vi "Results_Row_Per_Channel.vi"(0 "Analysis_info_cluster":T1={"Colour"=0, "Inst type"=enum."Pitot-static tube", "Inst name"="Manometer voltage", "Symbol"="U", "Code name"="", "Extra Info"="U", "Inst Array"=enum."PWA", "Extra Titles"=[], "Extra Values"=[], "U"=0.0, "u^2"=0.0, "u^3"=0.0, "u^4"=0.0, "Skew_u"=0.0, "Kurt_u"=0.0, "Sd Error in Mean"=0.0, "% u'/U"=0.0, "X"=0.0, "Y"=0.0, "Z"=0.0, "Timescale integral to 25%"=0.0, "Sd Error in Variance"=0.0, "Calib File"=path "", "Calib Constants"=[], "Output Position"=FALSE, "Full Stats"=FALSE, "Av Sampling Rate"=0.0, "Av No of Samples"=0.0, "Total Meas Time (s)"=0.0, "ADAM Ch Name"=""} {"Sd Error in Variance" format="%.2f"; "Skew_u" format="%.2f"; "% u'/U" format="%.2f"; "Sd Error in Mean" format="%.2f"; "Kurt_u" format="%.2f"; "u^4" format="%.2f"; "u^3" format="%.2f"; "U" format="%.2f"; "u^2" format="%.2f"}) -> (1 "Channel Names":string[](array[string]), 2 "Channel Values":string[](array[string]))   [LabVIEW 2014]
uses:
  Controls/Analysis_info_cluster.ctl
  Controls/Inst_type.ctl
  Controls/Instrument_Array.ctl
  Controls/Post_Process.ctl
  Globals/Trav_pos_global.vi
  Acquisition/PWA/PWAtasksGLOBAL.vi
  Globals/Meas_global.vi
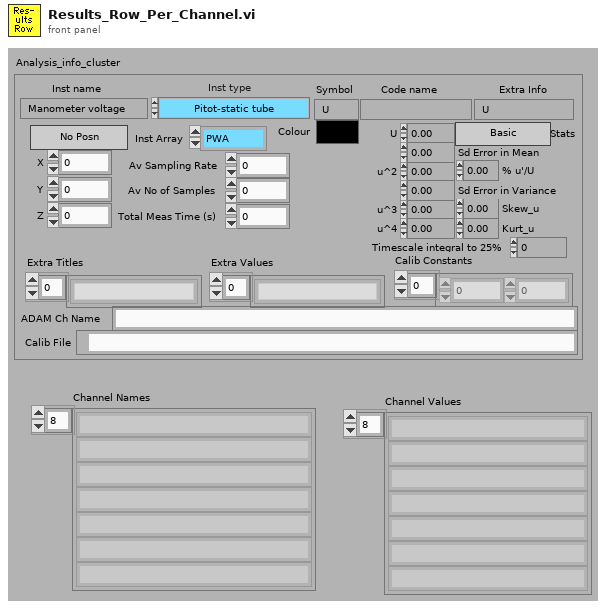
[diagram p1: front panel]
types:
  T1 = typedef "Analysis_info_cluster.ctl" = cluster{"Colour":u32, "Inst type":T2, "Inst name":string, "Symbol":string, "Code name":string, "Extra Info":string, "Inst Array":T3, "Extra Titles":string[], "Extra Values":string[], "U":dbl, "u^2":dbl, "u^3":dbl, "u^4":dbl, "Skew_u":dbl, "Kurt_u":dbl, "Sd Error in Mean":dbl, "% u'/U":dbl, "X":dbl, "Y":dbl, "Z":dbl, "Timescale integral to 25%":dbl, "Sd Error in Variance":dbl, "Calib File":path, "Calib Constants":dbl[], "Output Position":bool, "Full Stats":bool, "Av Sampling Rate":dbl, "Av No of Samples":dbl, "Total Meas Time (s)":dbl, "ADAM Ch Name":string}
  T2 = typedef "Inst_type.ctl" = enum16{"Propeller anemometer", "Raw voltage", "Pressure Transducer", "Pitot-static tube", "Preston tube", "Hot wire", "Cross wire 1", "Cross wire 2", "Generic Linear", "Generic Polynomial", "Generic BackPoly", "Fast FID", "Thermocouple", "Cold wire", "Pulsed Wire", "LDA Vel", "LDA Tran time", "LDA Arr time", "Microphone"}
  T3 = typedef "Instrument_Array.ctl" = enum16{"PWA", "LDA", "Analogue"}
  T4 = enum16{"Mean only", "2nd Order Stats", "4th Order Stats"}
  T5 = typedef "Post_Process.ctl" = enum16{"Take New Data", "Post Process Raw Data File"}
  T6 = typedef "Tunnel_Coordinates.ctl" = enum16{"Work in Tunnel Coordinates", "Work in Model Coordinates"}
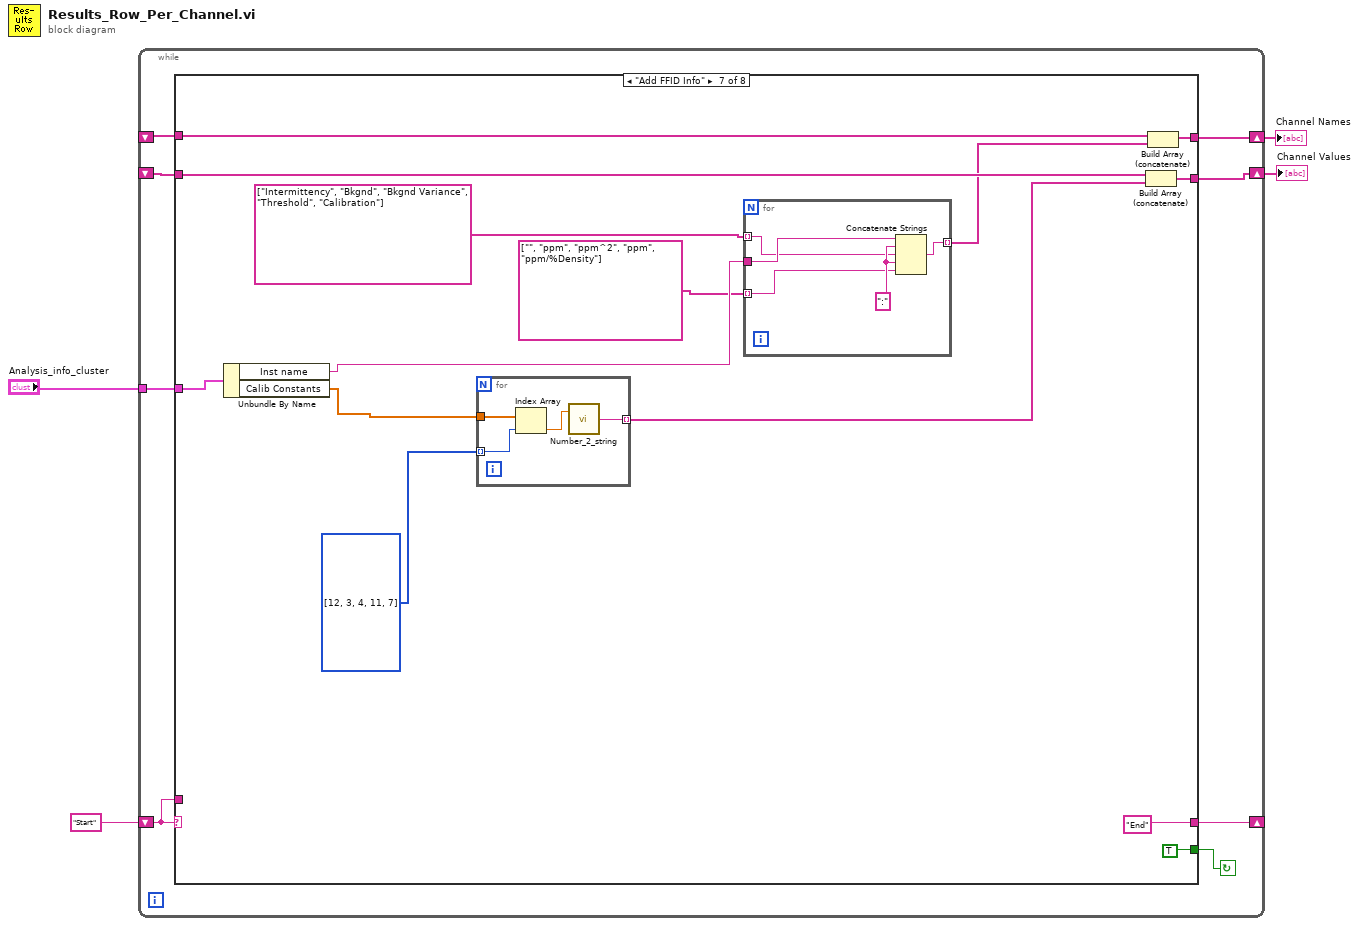
[diagram p0: block diagram]
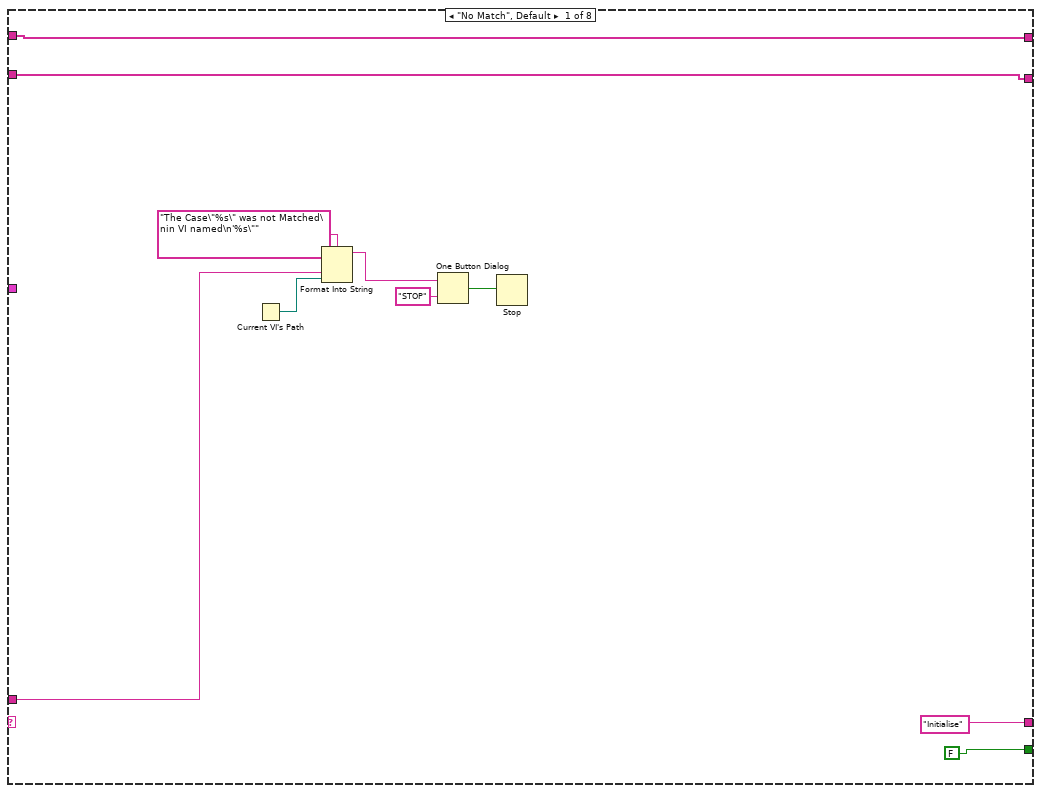
[diagram p2: hidden frame]
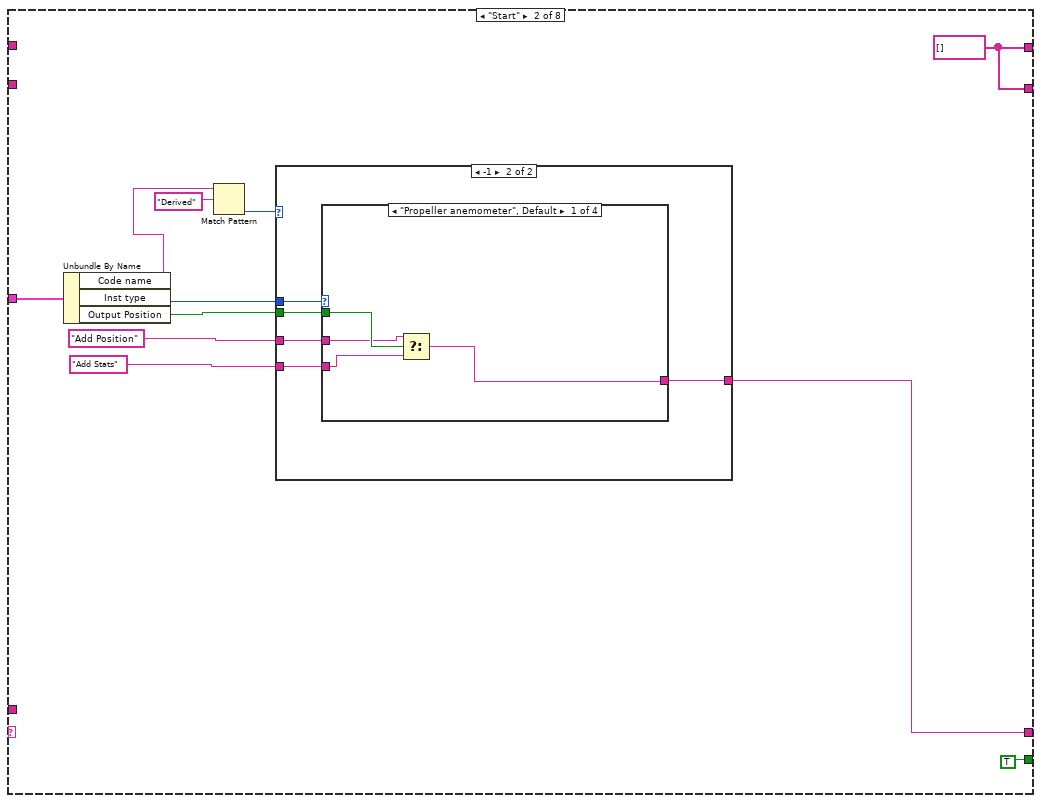
[diagram p3: hidden frame]
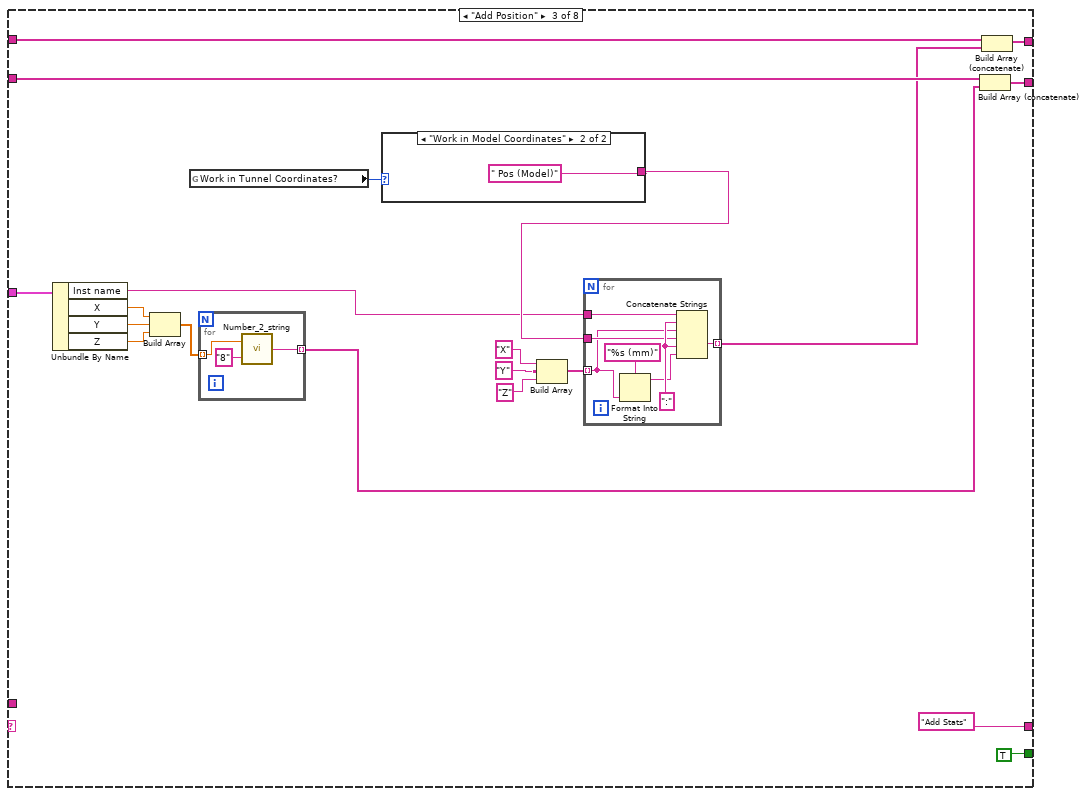
[diagram p8: hidden frame]
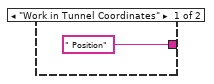
[diagram p9: hidden frame]
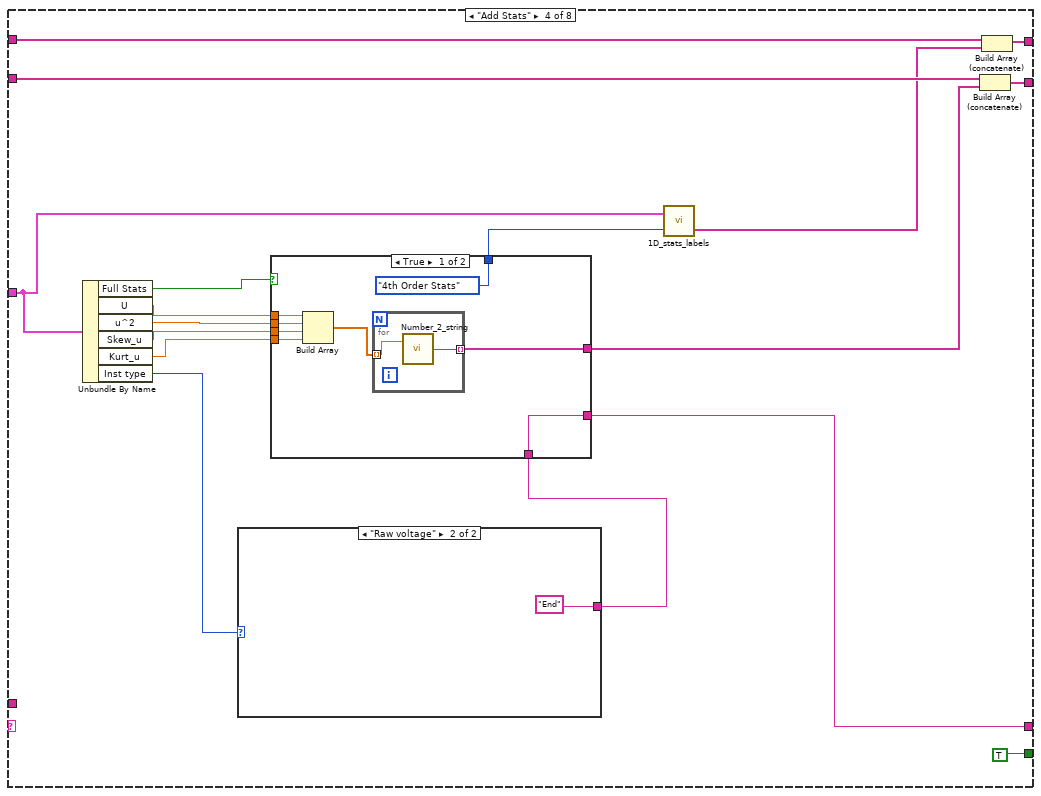
[diagram p10: hidden frame]
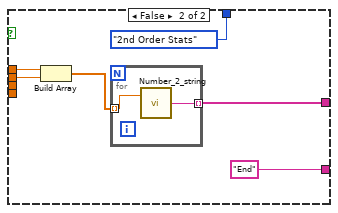
[diagram p11: hidden frame]
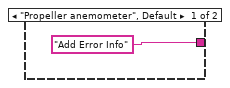
[diagram p12: hidden frame]
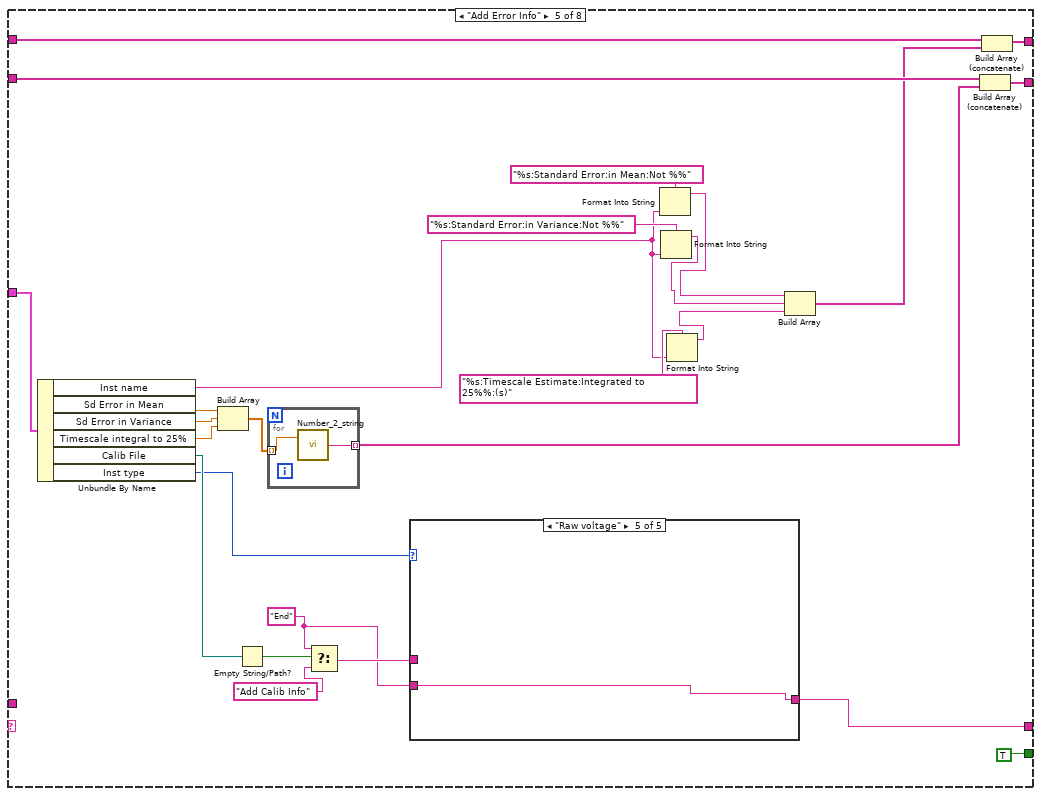
[diagram p13: hidden frame]
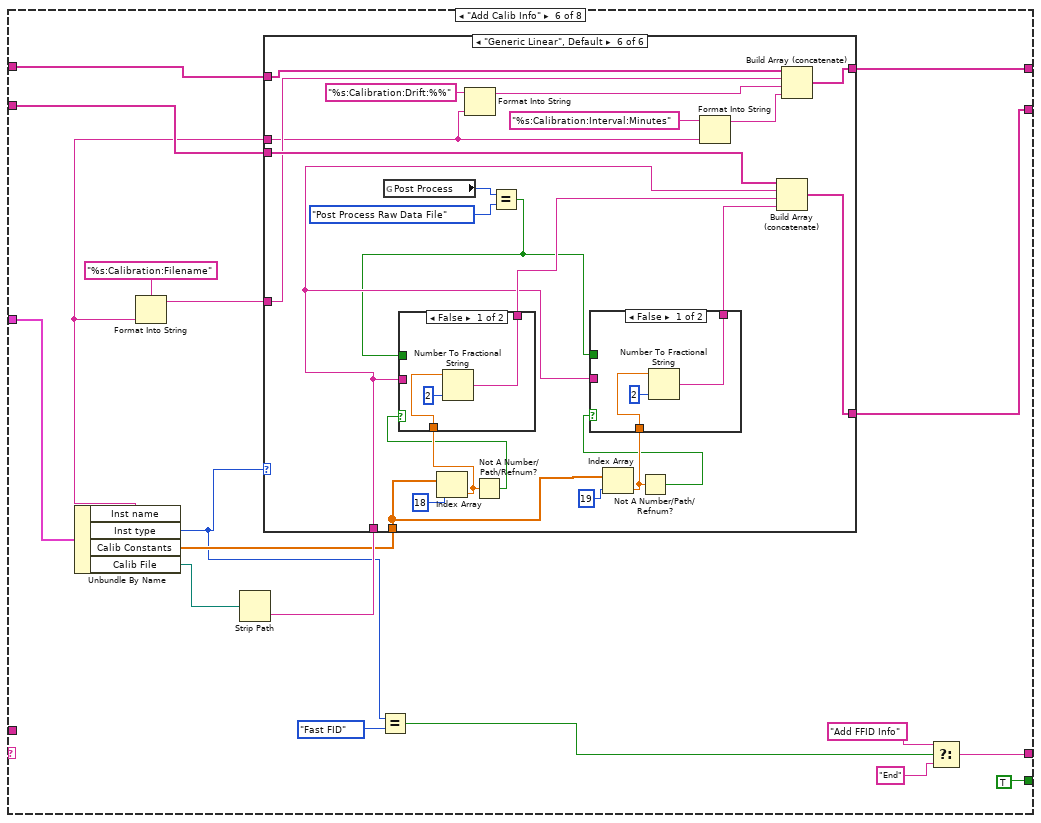
[diagram p18: hidden frame]
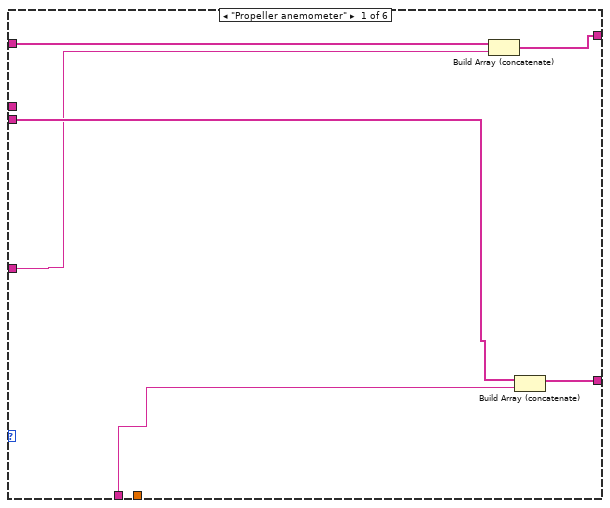
[diagram p19: hidden frame]
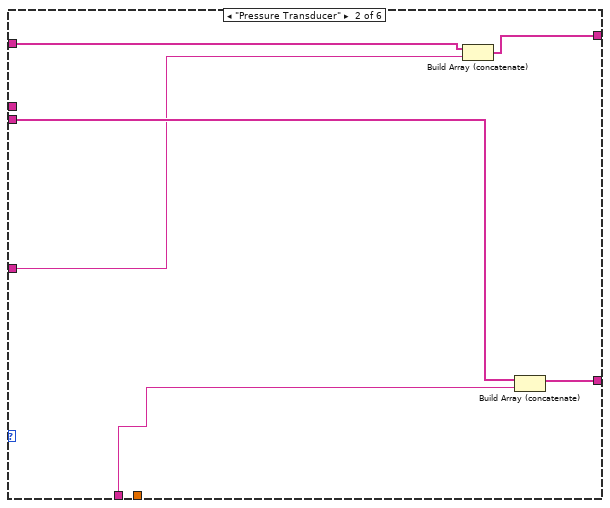
[diagram p20: hidden frame]
diagram:
  n1 = while {
    shift-left: "Start" -> [w10]
    shift-right: [w11] -> _
    shift-right: [w5] -> w1
    shift-left: _ -> [w6]
    shift-right: [w8] -> w2
    shift-left: _ -> [w7]
    tunnel: "Analysis_info_cluster" -> [w9]
    stop <- w12 continue-if-true
    n2 = case shown="\"Add FFID Info\"" w10 {
      tunnel: [FALSE TRUE TRUE TRUE TRUE TRUE TRUE FALSE] -> w12
      tunnel: ["Initialise" w30 "Add Stats" w81 w118 w151 "End" "End"] -> w11
      tunnel: w10 -> [w18 _ _ _ _ _ _ _]
      tunnel: w9 -> [_ w32 w58 w86 w133 w165 w247 w268]
      tunnel: [w13 w28 w51 w91 w137 w161 w251 w262] -> w8
      tunnel: w7 -> [w13 _ w50 w90 w136 w163 w250 w265]
      tunnel: w6 -> [w14 _ w49 w89 w135 w158 w249 w267]
      tunnel: [w14 w28 w48 w88 w134 w156 w248 w263] -> w5
      frame "No Match", Default {
        n3 = Current VI's Path() -> (path=w17:path)
        n4 = Format Into String(format string="The Case\"%s\" was not Matched\nin VI named\n'%s\"" ("Format String"), w18, w17) -> (resulting string=w21:string)  [unwired: 2 in, 1 out]
        n5 = One Button Dialog(message=w21, button name ("OK")="STOP") -> (true=w19:bool)
        n6 = Stop(stop? (T)=w19) -> ()
      }
      frame "Start" {
        w28 = string[] []
        n7 = Unbundle By Name(w32) -> ("Code name"=w25:string, "Inst type"=w31:T2, "Output Position"=w23:bool)
        n8 = Match Pattern(string=w25, regular expression="Derived") -> (offset past match=w24:i32)  [unwired: 1 in, 3 out]
        n9 = case shown="-1" w24 {
          tunnel: w31 -> [_ w39]
          tunnel: [w34 w38] -> w30
          tunnel: "Add Position" -> [_ w37]
          tunnel: "Add Stats" -> [w34 w36]
          tunnel: w23 -> [_ w35]
          frame 0, Default {
          }
          frame -1 {
            n10 = case shown="\"Propeller anemometer\", Default" w39 {
              tunnel: [w40 w44 w45 w46] -> w38
              tunnel: w37 -> [w42 _ _ _]
              tunnel: w36 -> [w41 w44 w45 w46]
              tunnel: w35 -> [w43 _ _ _]
              frame "Propeller anemometer", Default {
                n11 = Select(t=w42, s=w43, f=w41) -> (s? t:f=w40:string)
              }
              frame "Cross wire 2" {
              }
              frame "LDA Tran time" {
              }
              frame "LDA Arr time" {
              }
            }
          }
        }
      }
      frame "Add Position" {
        n12 = Unbundle By Name(w58) -> ("Inst name"=w57:string, "X"=w56:dbl, "Y"=w55:dbl, "Z"=w54:dbl)
        n13 = Build Array(w56, w55, w54) -> (w53:dbl[])
        n14 = global read "Trav_pos_global.vi" "Work in Tunnel Coordinates?"() -> (w64:T6)
        n15 = for {
          tunnel: w53 -> [w69] mode=indexing
          tunnel: [w68] -> w52 mode=indexing
          n16 = call "Number_2_string.vi"("precision"="8", "number"=w69) -> ("String"=w68:string)
        }
        n17 = case shown="\"Work in Model Coordinates\"" w64 {
          tunnel: [" Position" " Pos (Model)"] -> w59
          frame "Work in Tunnel Coordinates" {
          }
          frame "Work in Model Coordinates" {
          }
        }
        n18 = Build Array("X", "Y", "Z") -> (w63:string[])
        n19 = for {
          tunnel: w63 -> [w72] mode=indexing
          tunnel: w57 -> [w76]
          tunnel: [w74] -> w47 mode=indexing
          tunnel: w59 -> [w73]
          w75 = ":" ("Substring")
          n20 = Format Into String(format string="%s (mm)", w72) -> (resulting string=w70:string)  [unwired: 2 in, 1 out]
          n21 = Concatenate Strings(w76, w75, w72, w73, w75, w70) -> (w74:string)
        }
        n22 = Build Array (concatenate)(w50, w52) -> (w51:string[])
        n23 = Build Array (concatenate)(w49, w47) -> (w48:string[])
      }
      frame "Add Stats" {
        n24 = Unbundle By Name(w86) -> ("Full Stats"=w79:bool, "U"=w95:dbl, "u^2"=w94:dbl, "Skew_u"=w93:dbl, "Kurt_u"=w87:dbl, "Inst type"=w84:T2)
        n25 = case shown="\"Raw voltage\"" w84 {
          tunnel: ["Add Error Info" "End"] -> w80
          frame "Propeller anemometer", Default {
          }
          frame "Raw voltage" {
          }
        }
        n26 = case shown="True" w79 {
          tunnel: w95 -> [w103 w111]
          tunnel: w94 -> [w102 w110]
          tunnel: w93 -> [w101 _]
          tunnel: [w99 w108] -> w92
          tunnel: w87 -> [w98 _]
          tunnel: [T4."4th Order Stats" ("Mode selector") T4."2nd Order Stats" ("Mode selector")] -> w82
          tunnel: [w96 "End"] -> w81
          tunnel: w80 -> [w96 _]
          frame True {
            n27 = Build Array(w103, w102, w101, w98) -> (w100:dbl[])
            n28 = for {
              tunnel: w100 -> [w105] mode=indexing
              tunnel: [w104] -> w99 mode=indexing
              n29 = call "Number_2_string.vi"("number"=w105) -> ("String"=w104:string)  [unwired: 1 in]
            }
          }
          frame False {
            n30 = Build Array(w111, w110) -> (w109:dbl[])
            n31 = for {
              tunnel: w109 -> [w113] mode=indexing
              tunnel: [w112] -> w108 mode=indexing
              n32 = call "Number_2_string.vi"("number"=w113) -> ("String"=w112:string)  [unwired: 1 in]
            }
          }
        }
        n33 = call "1D_stats_labels.vi"("Mode selector"=w82, "Analysis Info Cluster"=w86) -> ("Output"=w85:string[])  [unwired: 1 in]
        n34 = Build Array (concatenate)(w90, w92) -> (w91:string[])
        n35 = Build Array (concatenate)(w89, w85) -> (w88:string[])
      }
      frame "Add Error Info" {
        w116 = "End"
        n36 = Unbundle By Name(w133) -> ("Inst name"=w126:string, "Sd Error in Mean"=w140:dbl, "Sd Error in Variance"=w124:dbl, "Timescale integral to 25%"=w123:dbl, "Calib File"=w122:path, "Inst type"=w117:T2)
        n37 = Build Array(w140, w124, w123) -> (w139:dbl[])
        n38 = Empty String/Path?(string/path=w122) -> (empty?=w121:bool)
        n39 = for {
          tunnel: w139 -> [w148] mode=indexing
          tunnel: [w147] -> w138 mode=indexing
          n40 = call "Number_2_string.vi"("number"=w148) -> ("String"=w147:string)  [unwired: 1 in]
        }
        n41 = Select(t=w116, s=w121, f="Add Calib Info") -> (s? t:f=w119:string)
        n42 = case shown="\"Raw voltage\"" w117 {
          tunnel: [w142 w143 w144 w145 w146] -> w118
          tunnel: w119 -> [w142 _ _ _ _]
          tunnel: w116 -> [_ w143 w144 w145 w146]
          frame "Propeller anemometer", Default {
          }
          frame "Cross wire 2" {
          }
          frame "LDA Tran time" {
          }
          frame "LDA Arr time" {
          }
          frame "Raw voltage" {
          }
        }
        n43 = Format Into String(format string="%s:Standard Error:in Mean:Not %%", w126) -> (resulting string=w128:string)  [unwired: 2 in, 1 out]
        n44 = Format Into String(format string="%s:Standard Error:in Variance:Not %%", w126) -> (resulting string=w130:string)  [unwired: 2 in, 1 out]
        n45 = Format Into String(format string="%s:Timescale Estimate:Integrated to 25%%:(s)", w126) -> (resulting string=w132:string)  [unwired: 2 in, 1 out]
        n46 = Build Array(w128, w130, w132) -> (w125:string[])
        n47 = Build Array (concatenate)(w136, w138) -> (w137:string[])
        n48 = Build Array (concatenate)(w135, w125) -> (w134:string[])
      }
      frame "Add Calib Info" {
        n49 = Unbundle By Name(w165) -> ("Inst name"=w155:string, "Inst type"=w154:T2, "Calib Constants"=w160:dbl[], "Calib File"=w164:path)
        n50 = Format Into String(format string="%s:Calibration:Filename" ("Format String"), w155) -> (resulting string=w157:string)  [unwired: 2 in, 1 out]
        n51 = Strip Path(path=w164) -> (name=w162:string)  [unwired: 1 out]
        n52 = case shown="\"Generic Linear\", Default" w154 {
          tunnel: [w172 w177 w183 w189 w196 w219] -> w161
          tunnel: w163 -> [w170 w178 w184 w190 w197 w220]
          tunnel: w162 -> [w171 w176 w182 w188 _ w213]
          tunnel: w160 -> [_ _ _ _ _ w212]
          tunnel: w158 -> [w169 w175 w181 w187 w193 w205]
          tunnel: w157 -> [w167 w174 w179 w186 w191 w204]
          tunnel: [w168 w173 w180 w185 w192 w199] -> w156
          tunnel: w155 -> [_ _ _ _ _ w198]
          frame "Propeller anemometer" {
            n53 = Build Array (concatenate)(w169, w167) -> (w168:string[])
            n54 = Build Array (concatenate)(w170, w171) -> (w172:string[])
          }
          frame "Pressure Transducer" {
            n55 = Build Array (concatenate)(w175, w174) -> (w173:string[])
            n56 = Build Array (concatenate)(w178, w176) -> (w177:string[])
          }
          frame "Pitot-static tube" {
            n57 = Build Array (concatenate)(w181, w179) -> (w180:string[])
            n58 = Build Array (concatenate)(w184, w182) -> (w183:string[])
          }
          frame "Preston tube" {
            n59 = Build Array (concatenate)(w190, w188) -> (w189:string[])
            n60 = Build Array (concatenate)(w187, w186) -> (w185:string[])
          }
          frame "Pulsed Wire" {
            n61 = global read "PWAtasksGLOBAL.vi" "PWA Calib. File Path"() -> (w195:path)
            n62 = Strip Path(path=w195) -> (name=w194:string)  [unwired: 1 out]
            n63 = Build Array (concatenate)(w193, w191) -> (w192:string[])
            n64 = Build Array (concatenate)(w197, w194) -> (w196:string[])
          }
          frame "Generic Linear", Default {
            n65 = global read "Meas_global.vi" "Post Process"() -> (w215:T5)
            n66 = Index Array(array=w212, index=18 ("Index")) -> (element=w218:dbl)
            n67 = Format Into String(format string="%s:Calibration:Drift:%%" ("Format String"), w198) -> (resulting string=w201:string)  [unwired: 2 in, 1 out]
            n68 = Not A Number/Path/Refnum?(number/path/refnum=w218) -> (NaN/Path/Refnum?=w217:bool)
            n69 = Equal?(x=w215, y=Post_Process."Post Process Raw Data File" ("Post Process")) -> (x = y?=w208:bool)
            n70 = case shown="False" w217 {
              tunnel: [w230 w235] -> w214
              tunnel: w218 -> [w231 _]
              tunnel: w208 -> [_ w237]
              tunnel: w213 -> [_ w234]
              frame False {
                n71 = Number To Fractional String(number=w231, precision (6)=i16 2) -> (F-format string=w230:string)  [unwired: 2 out]
              }
              frame True {
                n72 = Concatenate Strings(w234, "_Drift_Place_Holder" ("Substring")) -> (w236:string)
                n73 = Select(t="No Info", s=w237, f=w236) -> (s? t:f=w235:string)
              }
            }
            n74 = Index Array(array=w212, index=19 ("Index")) -> (element=w211:dbl)
            n75 = Not A Number/Path/Refnum?(number/path/refnum=w211) -> (NaN/Path/Refnum?=w210:bool)
            n76 = case shown="False" w210 {
              tunnel: [w221 w226] -> w209
              tunnel: w211 -> [w222 _]
              tunnel: w208 -> [_ w228]
              tunnel: w213 -> [_ w225]
              frame False {
                n77 = Number To Fractional String(number=w222, precision (6)=i16 2) -> (F-format string=w221:string)  [unwired: 2 out]
              }
              frame True {
                n78 = Concatenate Strings(w225, "_Interval_Place_Holder" ("Substring")) -> (w227:string)
                n79 = Select(t="No Info", s=w228, f=w227) -> (s? t:f=w226:string)
              }
            }
            n80 = Format Into String(format string="%s:Calibration:Interval:Minutes" ("Format String"), w198) -> (resulting string=w200:string)  [unwired: 2 in, 1 out]
            n81 = Build Array (concatenate)(w220, w213, w214, w209) -> (w219:string[])
            n82 = Build Array (concatenate)(w205, w204, w201, w200) -> (w199:string[])
          }
        }
        n83 = Equal?(x=w154, y=Inst_type."Fast FID" ("Inst type")) -> (x = y?=w153:bool)
        n84 = Select(t="Add FFID Info", s=w153, f="End") -> (s? t:f=w151:string)
      }
      frame "Add FFID Info" {
        n85 = Unbundle By Name(w247) -> ("Inst name"=w242:string, "Calib Constants"=w245:dbl[])
        n86 = for {
          tunnel: w245 -> [w261]
          tunnel: i32[] [12, 3, 4, 11, 7] ("Calib Constants") -> [w260] mode=indexing
          tunnel: [w258] -> w243 mode=indexing
          n87 = Index Array(array=w261, index=w260) -> (element=w259:dbl)
          n88 = call "Number_2_string.vi"("number"=w259) -> ("String"=w258:string)  [unwired: 1 in]
        }
        n89 = for {
          tunnel: string[] ["Intermittency", "Bkgnd", "Bkgnd Variance", "Threshold", "Calibration"] ("appended array") -> [w254] mode=indexing
          tunnel: w242 -> [w255]
          tunnel: [w256] -> w241 mode=indexing
          tunnel: string[] ["", "ppm", "ppm^2", "ppm", "ppm/%Density"] ("appended array") -> [w253] mode=indexing
          w257 = ":" ("Substring")
          n90 = Concatenate Strings(w255, w257, w254, w257, w253) -> (w256:string)
        }
        n91 = Build Array (concatenate)(w250, w243) -> (w251:string[])
        n92 = Build Array (concatenate)(w249, w241) -> (w248:string[])
      }
      frame "End" {
        n93 = Unbundle By Name(w268) -> ("Extra Titles"=w266:string[], "Extra Values"=w264:string[])
        n94 = Build Array (concatenate)(w267, w266) -> (w263:string[])
        n95 = Build Array (concatenate)(w265, w264) -> (w262:string[])
      }
    }
  }
  "Channel Names" <- w1
  "Channel Values" <- w2
